vi "Measure Power.vi"(8 "error in":errorcluster, 10 "Channel":T1, 11 "2936r in":refnum<class "2936r.lvclass">) -> (0 "error out":errorcluster, 2 "Power Measured":dbl, 3 "2936r out":refnum<class "2936r.lvclass">)   [LabVIEW 2017, in "2936r.lvlib" / "2936r.lvclass"]
uses:
  2936r.lvclass
  builds/Optical Power Meter.lvlibp/Custom Controls/Channel List.ctl
  2936r.lvclass/2936r.ctl
  builds/Optical Power Meter.lvlibp
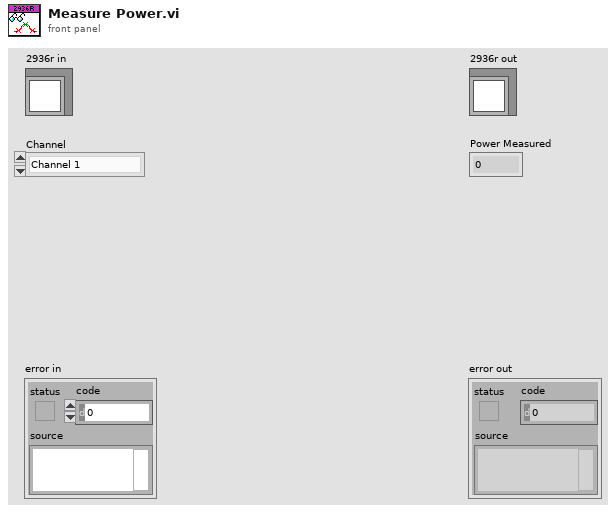
[diagram p1: front panel]
types:
  T1 = typedef "Optical Power Meter.lvlibp/Channel List.ctl" = enum16{"Channel 1", "Channel 2", "Channel 3", "Channel 4"}
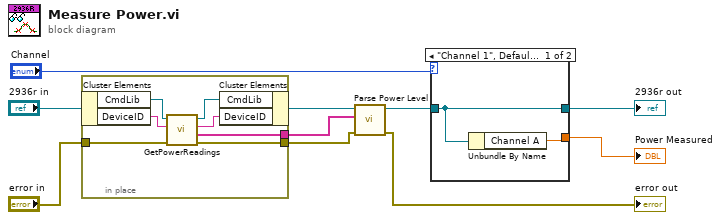
[diagram p0: block diagram]
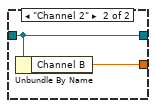
[diagram p2: hidden frame]
diagram:
  n1 = in-place {
    in-place-border: [w17] -> w10
    in-place-border: [w16] -> w9
    in-place-border: "error in" -> [w15]
    n2 = in-place-cluster #1("2936r in") -> ("CmdLib"=w14:refnum<k24>, "DeviceID"=w13:string)
    n3 = call <instrlib>:"GetPowerReadings.vi"("error in"=w15, "Device Key In"=w13, "PM Cmds In"=w14) -> ("error out"=w16:errorcluster, "Power Readings"=w17:string[], "Device Key Out"=w11:string, "PM Cmds Out"=w12:refnum<k24>)  [unwired: 1 in]
    n4 = in-place-cluster #1("CmdLib"=w12, "DeviceID"=w11) -> (w1:refnum<class "2936r.lvclass">)
  }
  n5 = call "Parse Power Level.vi"("error in"=w9, "Read Values"=w10, "2936r in"=w1) -> ("error out"=→"error out":errorcluster, "2936r out"=w7:refnum<class "2936r.lvclass">)  [unwired: 7 in]
  n6 = case shown="\"Channel 1\", Default" "Channel" {
    tunnel: w7 -> [w19 w21]
    tunnel: [w19 w21] -> w6
    tunnel: [w18 w20] -> w5
    frame "Channel 1", Default {
      n7 = Unbundle By Name(w19) -> ("Channel A"=w18:dbl)
    }
    frame "Channel 2" {
      n8 = Unbundle By Name(w21) -> ("Channel B"=w20:dbl)
    }
  }
  "2936r out" <- w6
  "Power Measured" <- w5
